vi "Ex5-v2-write-data.vi"() -> ()   [LabVIEW 2021]
uses:
  <vilib>/Utility/NIReport.llb/Report Type.ctl
  <vilib>/addons/_office/excel.llb/Excel Get Data ([str]).vi
  <vilib>/addons/_office/excel.llb/Excel Easy Table (str).vi
  <vilib>/Utility/NIReport.llb/NI_report.lvclass
  <vilib>/Utility/NIReport.llb/NI_ReportGenerationCore.lvlib
  <vilib>/addons/_office/NI_ReportGenerationToolkit.lvlib
  <vilib>/Utility/NIReport.llb/Excel/NI_Excel.lvclass
panel:
  in  "outside border":T1={"on/off"=TRUE, "weight"=2, "color"=13816530} {"weight" items=["xlHairline"=1, "xlMedium"=-4138, "xlThick"=4, "xlThin"=2]}
  in  "inside border":T1={"on/off"=TRUE, "weight"=2, "color"=13816530} {"weight" items=["xlHairline"=1, "xlMedium"=-4138, "xlThick"=4, "xlThin"=2]}
  in  "Save Button":bool
  in  "data":string[][](array[string])=[["1", "5.15491870640089"], ["2", "5.67423832036792"], ["3", "5.2163787188103"], ["4", "5.06029311600493"], ["5", "5.32744301432364"], ["6", "5.31183942496621"], ["7", "5.93093181517557"], ["8", "5.23183762963235"], ["9", "5.62991766337104"], ["10", "5.71484892598602"]]
  in  "Stop Button":bool
  in  "Text Ring":u16(ring)=6 items=["(5)", "(4)", "(3)", "(2)", "(1)", "Summary 1", "Data 2"]
  out "Sheet names":string[](array[string])=["(5)", "(4)", "(3)", "(2)", "(1)", "Summary 1", "Data 2"]
  out "error out":errorcluster
  in  "File Path":path=path "C:/Users/PLS_2/OneDrive/Desktop/LabVIEW with excel/mockup.xlsx"
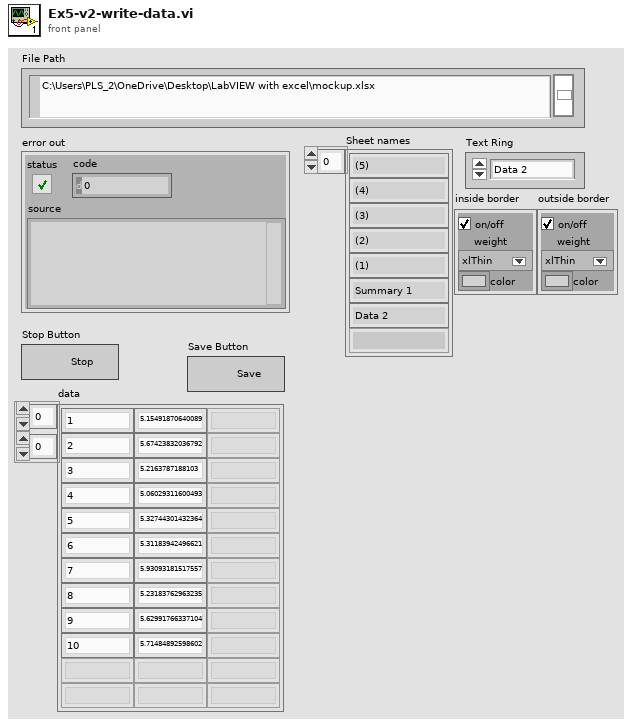
[diagram p1: front panel]
types:
  T1 = cluster{"on/off":bool, "weight":i32, "color":u32}
  T2 = typedef "NI_ReportGenerationCore.lvlib/Report Type.ctl" = enum16{"HTML", "Word", "Excel"}
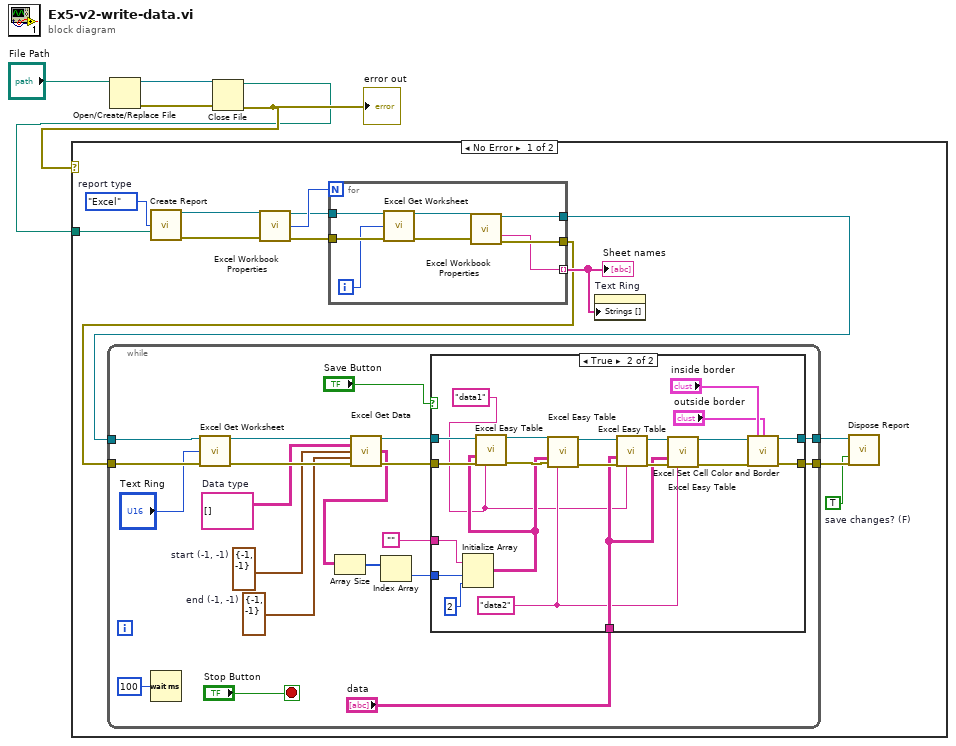
[diagram p0: block diagram]
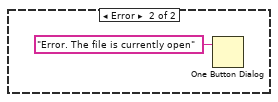
[diagram p3: hidden frame]
diagram:
  n1 = Open/Create/Replace File(file path (use dialog)="File Path") -> (refnum out=w5:refnum<file>, error out=w4:errorcluster)  [unwired: 5 in, 1 out]
  n2 = Close File(refnum=w5, error in=w4) -> (path=w1:path, error out=w3:errorcluster)
  "error out" <- w3
  n3 = case shown="No Error" w3 {
    tunnel: w1 -> [w18 _]
    frame No Error {
      w6 = TRUE  # save changes? (F)
      w17 = Report_Type."Excel"  # report type
      n4 = call <vilib>:"Create Report.vi"("report type"=w17, "template (empty)"=w18) -> ("report out"=w16:refnum<class "NI_report.lvclass">, "error out"=w15:errorcluster)  [unwired: 12 in]
      n5 = call <vilib>:"Excel Workbook Properties.vi"("report in"=w16, "error in (no error)"=w15) -> ("report out"=w13:refnum<class "NI_report.lvclass">, "worksheets count"=w14:i32, "error out"=w12:errorcluster)  [unwired: 10 in, 1 out]
      n6 = for {
        N: w14 -> [_]
        tunnel: w13 -> [w69]
        tunnel: w12 -> [w68]
        tunnel: [w64] -> w10
        tunnel: [w63] -> w9
        tunnel: [w62] -> w11 mode=indexing
        i -> [w67]
        n7 = call <vilib>:"Excel Get Worksheet.vi"("report in"=w69, "worksheet index (0)"=w67, "error in (no error)"=w68) -> ("report out"=w66:refnum<class "NI_report.lvclass">, "error out"=w65:errorcluster)  [unwired: 11 in]
        n8 = call <vilib>:"Excel Workbook Properties.vi"("report in"=w66, "error in (no error)"=w65) -> ("report out"=w64:refnum<class "NI_report.lvclass">, "current worksheet name"=w62:string, "error out"=w63:errorcluster)  [unwired: 10 in, 1 out]
      }
      "Sheet names" <- w11
      n9 = while {
        tunnel: w10 -> [w38]
        tunnel: w9 -> [w37]
        tunnel: [w26] -> w8
        tunnel: [w25] -> w7
        stop <- "Stop Button" stop-if-true
        w29 = cluster{"row":i32, "column":i32} {"row"=-1, "column"=-1}  # end (-1, -1)
        w30 = cluster{"row":i32, "column":i32} {"row"=-1, "column"=-1}  # start (-1, -1)
        w31 = string[][] []  # Data type
        n10 = Wait (ms)(milliseconds to wait=u32 100) -> ()  [unwired: 1 out]
        n11 = call <vilib>:"Excel Get Worksheet.vi"("report in"=w38, "worksheet index (0)"="Text Ring", "error in (no error)"=w37) -> ("report out"=w33:refnum<class "NI_report.lvclass">, "error out"=w32:errorcluster)  [unwired: 11 in]
        n12 = call-poly <vilib>:"Excel Get Data.vi"("report in"=w33, "data type"=w31, "start (-1, -1)"=w30, "end (-1, -1)"=w29, "error in (no error)"=w32) -> ("report out"=w28:refnum<class "NI_report.lvclass">, "data"=w22:string[][], "error out"=w27:errorcluster)  [unwired: 8 in]
        n13 = Array Size(array=w22) -> (size(s)=w21:i32[])
        n14 = Index Array(array=w21) -> (element=w20:i32)  [unwired: 1 in]
        n15 = case shown="True" "Save Button" {
          tunnel: w28 -> [w40 w48]
          tunnel: w27 -> [w39 w47]
          tunnel: [w40 w54] -> w26
          tunnel: [w39 w53] -> w25
          tunnel: "data" -> [_ w43]
          tunnel: w20 -> [_ w58]
          tunnel: "" -> [_ w57]
          frame False {
          }
          frame True {
            w41 = "data1" ("name (\"\")")
            w42 = "data2" ("name (\"\")")
            n16 = Initialize Array "Initialize Array"(w57, w58, 2 ("dimension size")) -> (w44:string[][])
            n17 = call-poly <vilib>:"Excel Easy Table.vi"("report in"=w48, "text data"=w44, "error in (no error)"=w47, "name (\"\")"=w41) -> ("report out"=w46:refnum<class "NI_report.lvclass">, "error out"=w45:errorcluster)  [unwired: 7 in, 3 out]
            n18 = call-poly <vilib>:"Excel Easy Table.vi"("report in"=w46, "text data"=w44, "error in (no error)"=w45, "name (\"\")"=w42) -> ("report out"=w61:refnum<class "NI_report.lvclass">, "error out"=w60:errorcluster)  [unwired: 7 in, 3 out]
            n19 = call-poly <vilib>:"Excel Easy Table.vi"("report in"=w61, "text data"=w43, "error in (no error)"=w60, "name (\"\")"=w41) -> ("report out"=w52:refnum<class "NI_report.lvclass">, "error out"=w51:errorcluster)  [unwired: 7 in, 3 out]
            n20 = call-poly <vilib>:"Excel Easy Table.vi"("report in"=w52, "text data"=w43, "error in (no error)"=w51, "name (\"\")"=w42) -> ("report out"=w50:refnum<class "NI_report.lvclass">, "error out"=w49:errorcluster)  [unwired: 7 in, 3 out]
            n21 = call <vilib>:"Excel Set Cell Color and Border.vi"("report in"=w50, "inside border"="inside border", "outside border"="outside border", "error in (no error)"=w49) -> ("report out"=w54:refnum<class "NI_report.lvclass">, "error out"=w53:errorcluster)  [unwired: 10 in]
          }
        }
      }
      n22 = property on="Text Ring" class="Ring (strict)"("Strings []"=w11) -> ()  [unwired: 2 in, 2 out]
      n23 = call-dynamic "Dispose Report.vi"("report in"=w8, "save changes? (F)"=w6, "error in (no error)"=w7) -> ()  [unwired: 12 in, 1 out]
    }
    frame Error {
      n24 = One Button Dialog(message="Error. The file is currently open") -> ()  [unwired: 1 in, 1 out]
    }
  }
